vi "subItemThird(json).vi"(4 "pointLimit":string, 6 "single frequency":string, 7 "single frequency value":string, 8 "single frequency result":string, 9 "SN":string, 10 "third test item name":string, 11 "subIDcount":i32) -> (2 "SubItem":string)   [LabVIEW 2011]
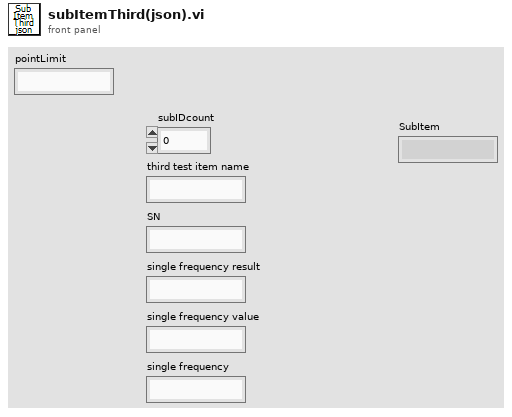
[diagram p1: front panel]
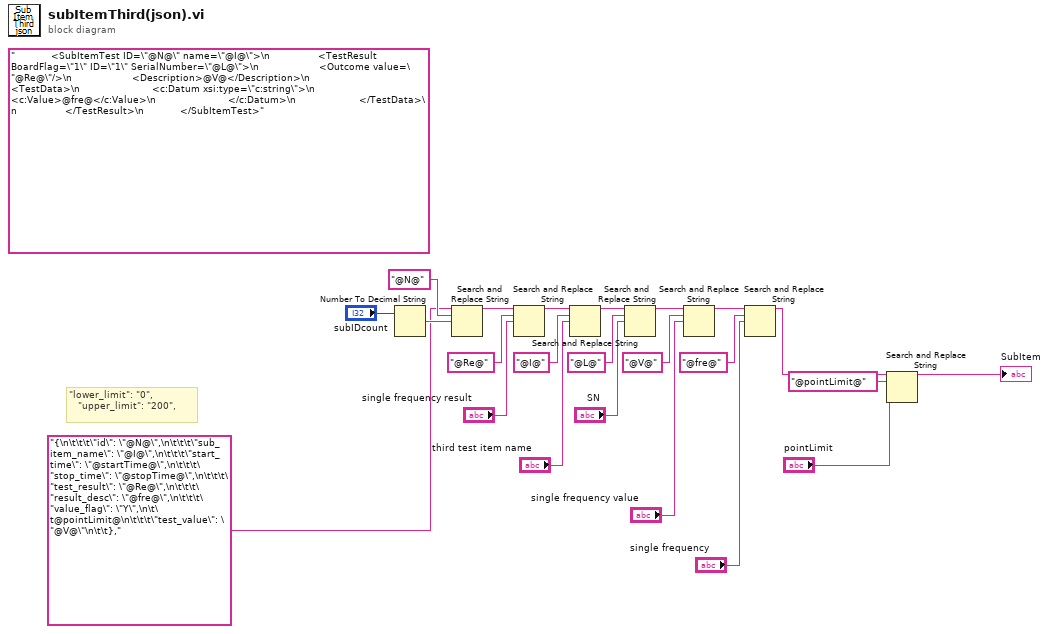
[diagram p0: block diagram]
diagram:
  (unwired) "            <SubItemTest ID=\"@N@\" name=\"@I@\">\n                <TestResult BoardFlag=\"1\" ID=\"1\" SerialNumber=\"@L@\">\n                    <Outcome value=\"@Re@\"/>\n                    <Description>@V@</Description>\n                    <TestData>\n                        <c:Datum xsi:type=\"c:string\">\n                            <c:Value>@fre@</c:Value>\n                        </c:Datum>\n                     </TestData>\n                </TestResult>\n            </SubItemTest>"
  # "\"lower_limit\": \"0\",\n\t\t\t\"upper_limit\": \"200\","
  n1 = Number To Decimal String(number="subIDcount") -> (decimal integer string=w22:string)  [unwired: 1 in]
  n2 = Search and Replace String(input string="{\n\t\t\t\"id\": \"@N@\",\n\t\t\t\"sub_item_name\": \"@I@\",\n\t\t\t\"start_time\": \"@startTime@\",\n\t\t\t\"stop_time\": \"@stopTime@\",\n\t\t\t\"test_result\": \"@Re@\",\n\t\t\t\"result_desc\": \"@fre@\",\n\t\t\t\"value_flag\": \"Y\",\n\t\t@pointLimit@\n\t\t\t\"test_value\": \"@V@\"\n\t\t},", search string="@N@" ("搜索字符串"), replace string=w22) -> (result string=w14:string)  [unwired: 5 in, 3 out]
  n3 = Search and Replace String(input string=w14, search string="@Re@" ("搜索字符串"), replace string="single frequency result") -> (result string=w12:string)  [unwired: 5 in, 3 out]
  n4 = Search and Replace String(input string=w12, search string="@I@" ("搜索字符串"), replace string="third test item name") -> (result string=w20:string)  [unwired: 5 in, 3 out]
  n5 = Search and Replace String(input string=w20, search string="@L@" ("搜索字符串"), replace string="SN") -> (result string=w17:string)  [unwired: 5 in, 3 out]
  n6 = Search and Replace String(input string=w17, search string="@V@" ("搜索字符串"), replace string="single frequency value") -> (result string=w16:string)  [unwired: 5 in, 3 out]
  n7 = Search and Replace String(input string=w16, search string="@fre@" ("搜索字符串"), replace string="single frequency") -> (result string=w4:string)  [unwired: 5 in, 3 out]
  n8 = Search and Replace String(input string=w4, search string="@pointLimit@" ("搜索字符串"), replace string="pointLimit") -> (result string=→"SubItem":string)  [unwired: 5 in, 3 out]
